vi "main.vi"() -> ()   [LabVIEW 2024]
uses:
  Controls/Who.ctl
  Controls/StratagemRing.ctl
  Controls/StateMachineState.ctl
  Controls/GameInfo.ctl
  Controls/E_Phases.ctl
  <vilib>/Platform/browser.llb/Open URL in Default Browser (string).vi
panel:
  in  "LastGame":bool
  in  "End Game":bool
  in  "Stratagems":T1 {"Cost" items=[" 1 CP", " 1 CP", " 2 CP", " 0 CP"]; "Name" items=["Command Reroll", " Smoke", " Fire and Fade", " Not in Data"]}
  in  "Spend2":bool
  in  "Spend1":bool
  in  "StratList":bool
  out "Wiki":string="Feeling lost? Click me to use Wiki "
  in  "DiscardM2":bool
  in  "DiscardM1":bool
  in  "Mission 2":dbl
  in  "Mission 1":dbl
  out "Victory points":dbl
  in  "Scored Primary":dbl
  out "BattleRound":dbl
  out "Command Points":dbl
  out "DidIStart?":bool
  in  "Who is going first?":T2
  out "Phase":string
  in  "GainCP":bool
  in  "NextPhase":bool
  in  "StartGame":bool
  out "error out":errorcluster
  in  "error in":errorcluster
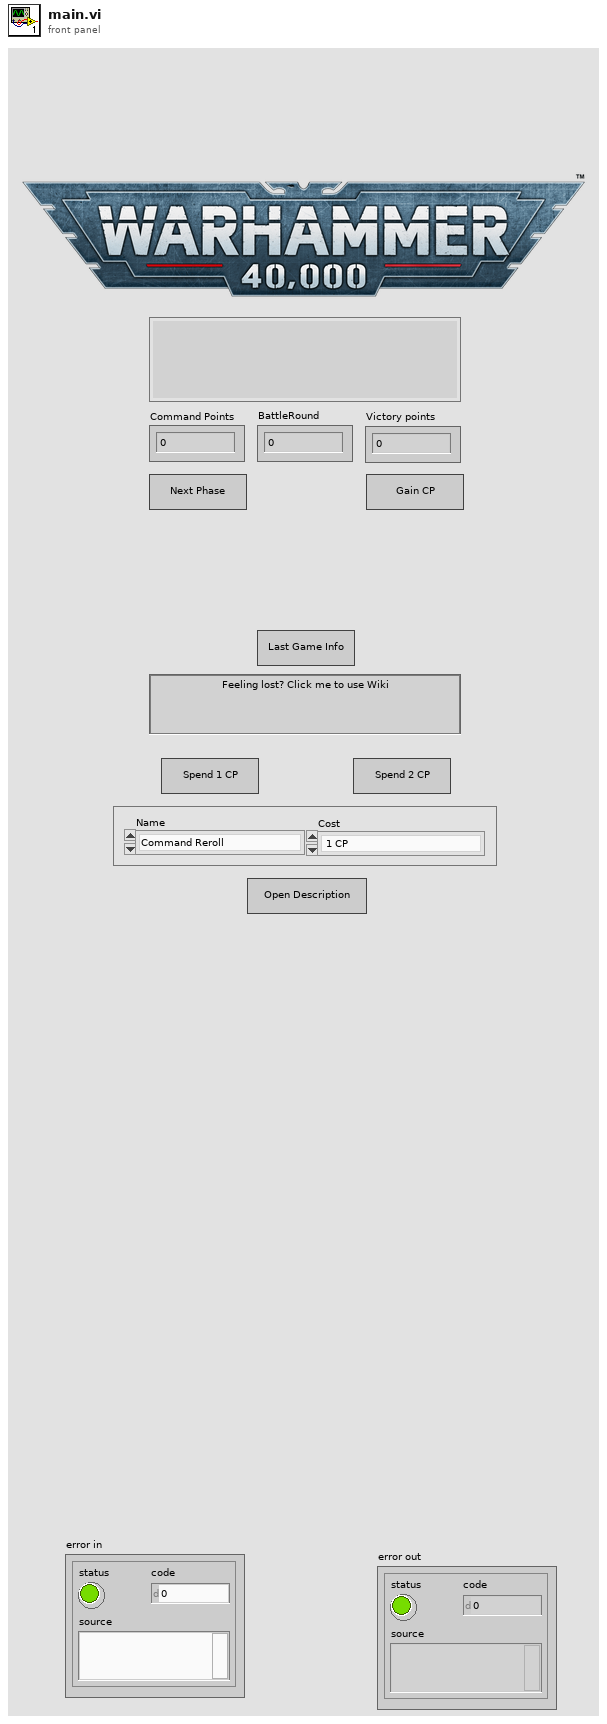
[diagram p1: front panel]
types:
  T1 = typedef "StratagemRing.ctl" = cluster{"Name":u16, "Cost":u16}
  T2 = typedef "Who.ctl" = enum16{"Me", "Opponent"}
  T3 = typedef "GameInfo.ctl" = cluster{"Player":string, "Opponent":string, "PArmy":string, "OArmy":string, "CP":dbl, "VP":dbl, "GameStart":timestamp, "GameEnd":timestamp, "BattleRound":dbl, "PrimaryMissionPoints":dbl, "SecondaryMissionPoints":dbl, "BattlePhase":T4, "Win":dbl, "Lose":dbl}
  T4 = typedef "E_Phases.ctl" = enum16{"Null/Error", "Command Phase", "Movement Phase", "Shooting Phase", "Charge Phase", "Fight Phase", "Secondary Scoring", "Enemy Command Phase", "Enemy Movement Phase", "Enemy Shooting Phase", "Enemy Charge Phase", "Enemy Fight Phase", "Enemy Secondary Scoring"}
  T5 = typedef "StateMachineState.ctl" = enum16{"Application Error", "Init", "Idle", "DataAnalysis", "Save", "Stop", "Error Handling"}
  T6 = enum8{"Enabled", "Disabled", "Disabled and Grayed Out"}
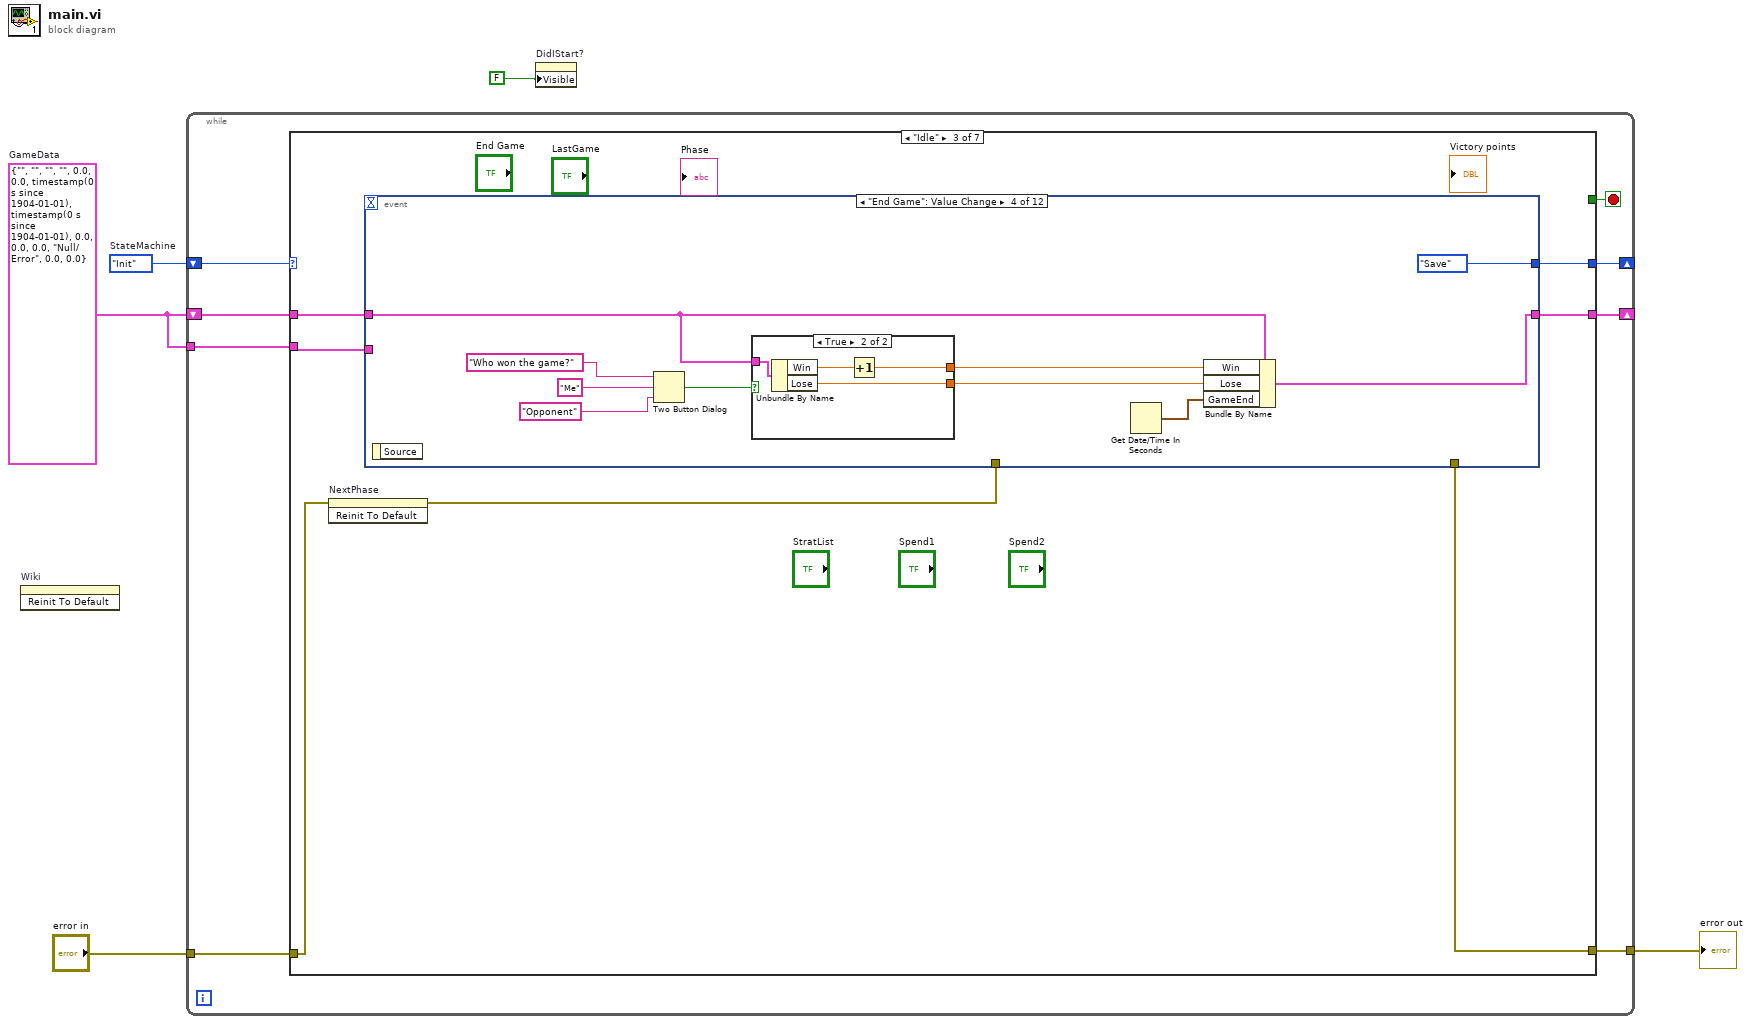
[diagram p0: block diagram]
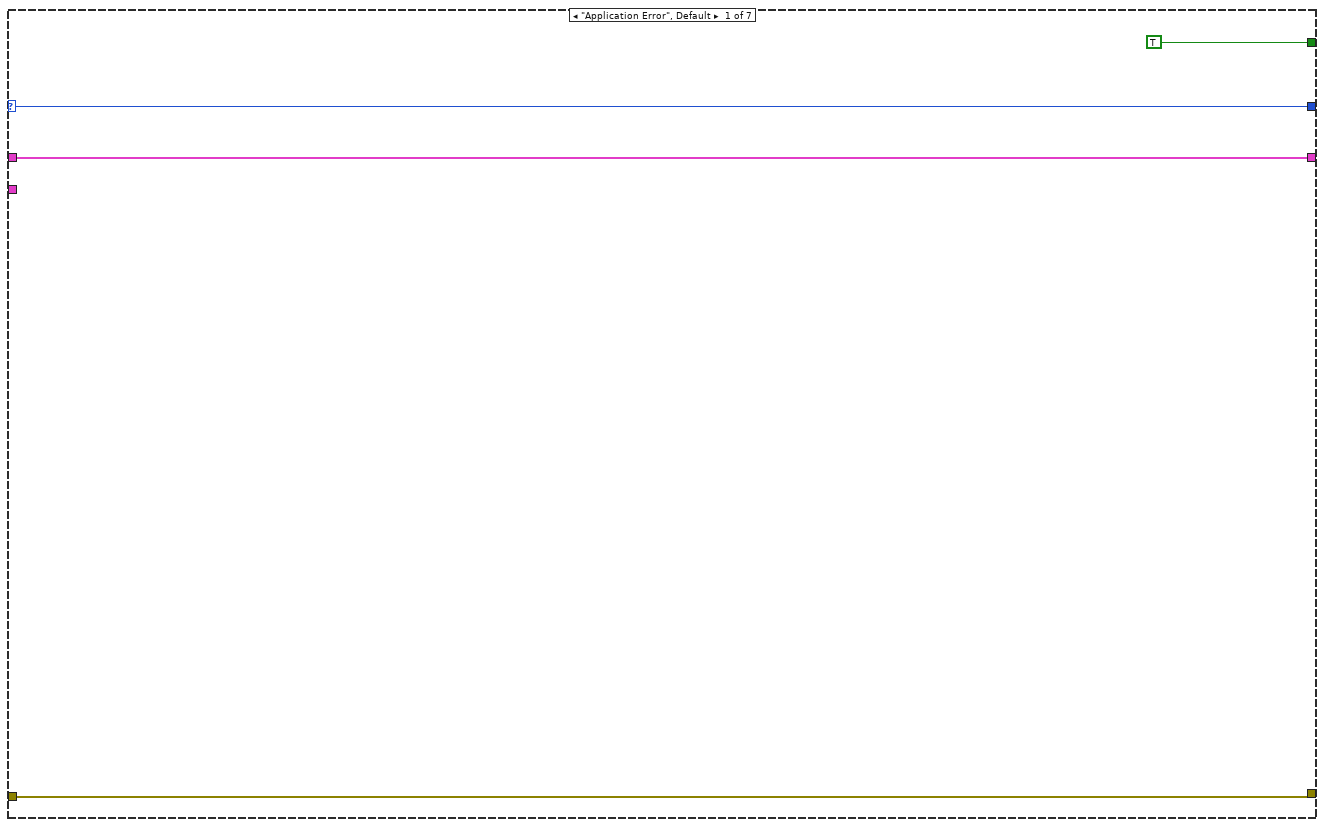
[diagram p2: hidden frame]
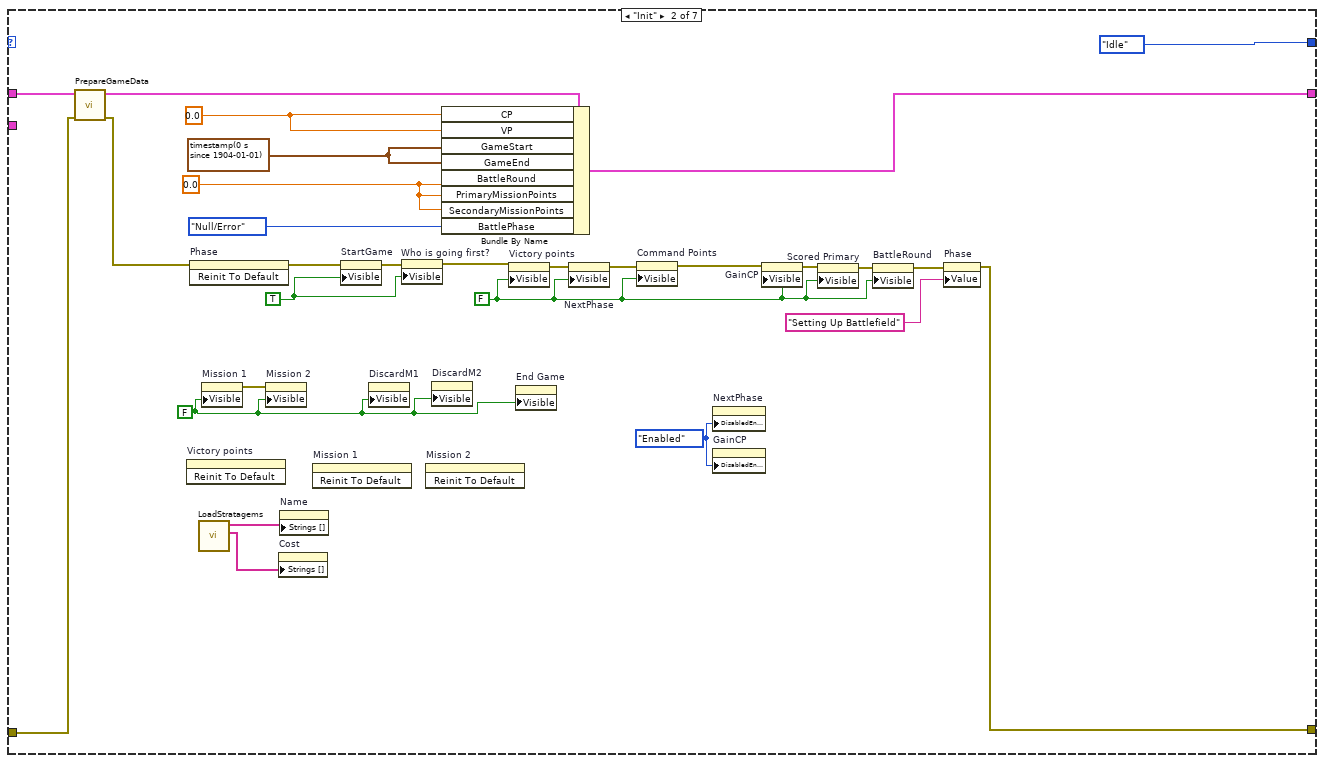
[diagram p3: hidden frame]
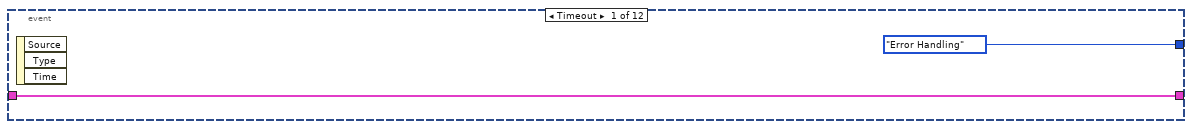
[diagram p4: hidden frame]
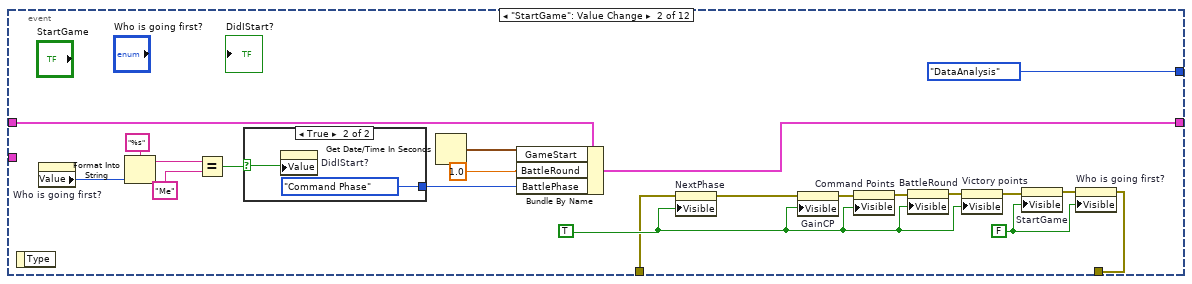
[diagram p5: hidden frame]
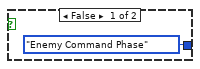
[diagram p6: hidden frame]
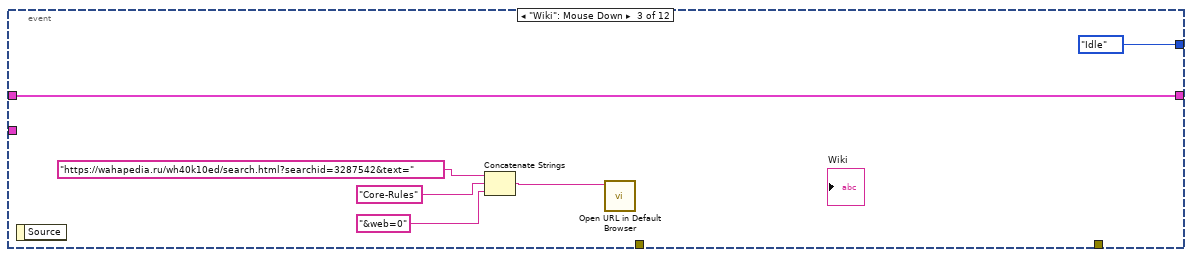
[diagram p7: hidden frame]
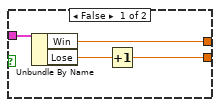
[diagram p8: hidden frame]
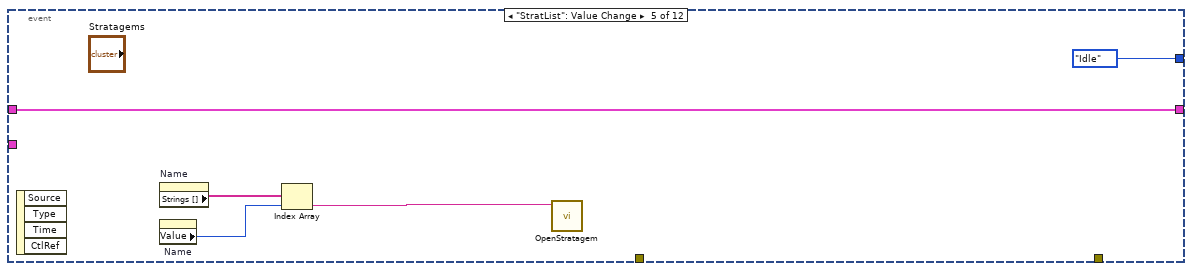
[diagram p9: hidden frame]
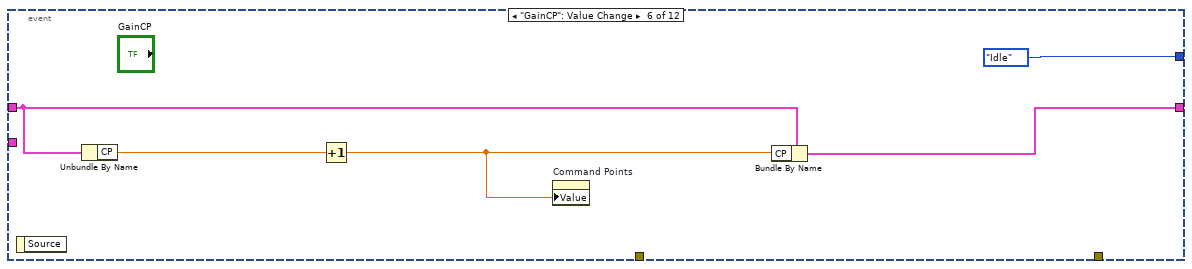
[diagram p10: hidden frame]
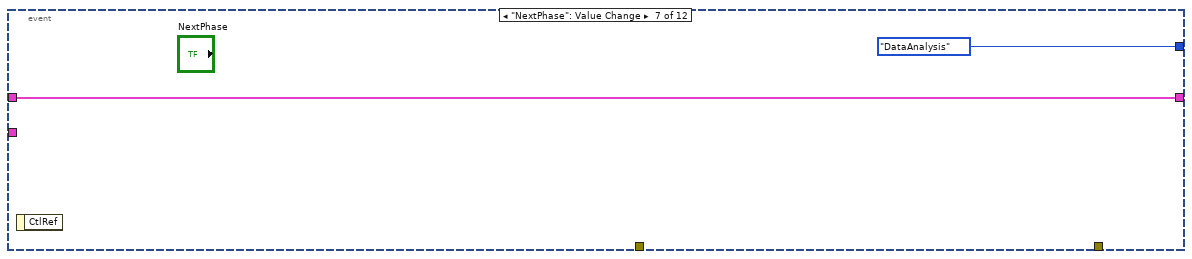
[diagram p11: hidden frame]
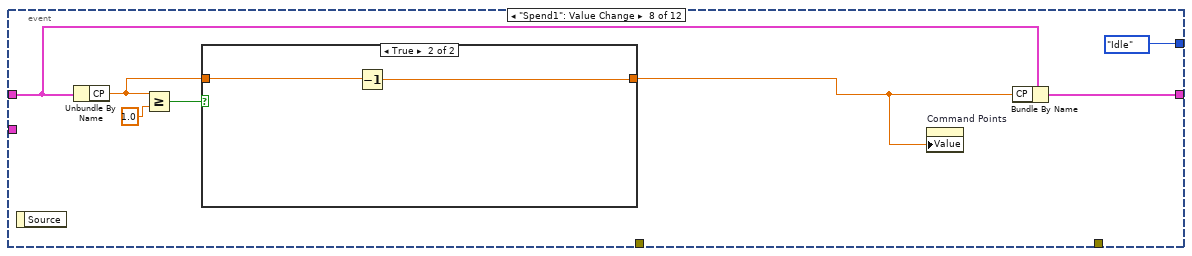
[diagram p12: hidden frame]
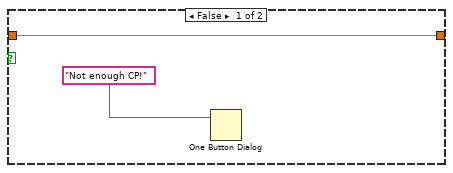
[diagram p13: hidden frame]
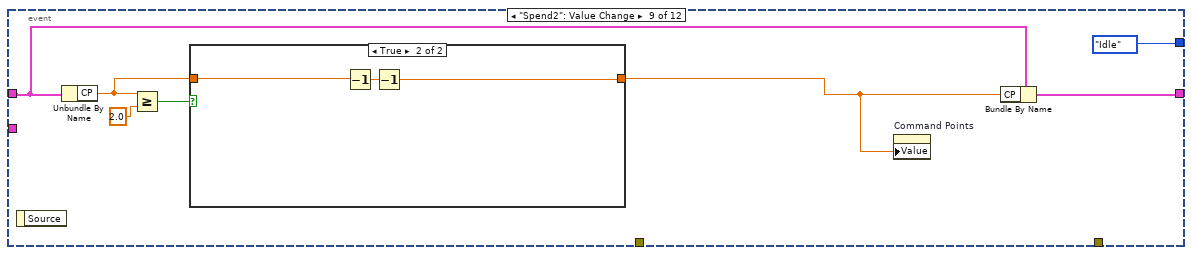
[diagram p14: hidden frame]
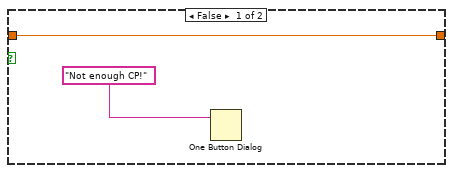
[diagram p15: hidden frame]
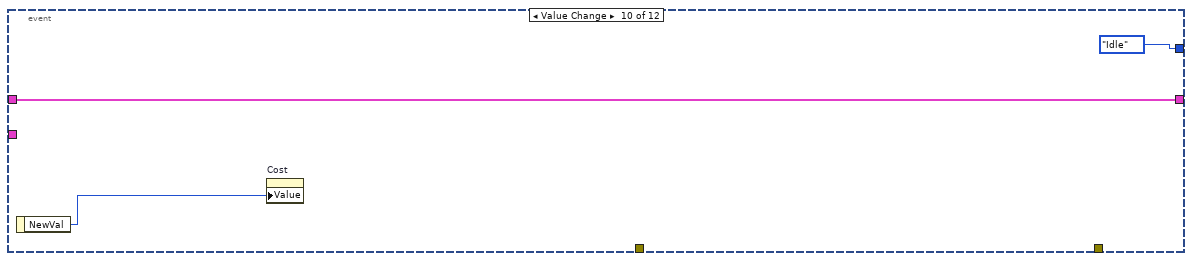
[diagram p16: hidden frame]
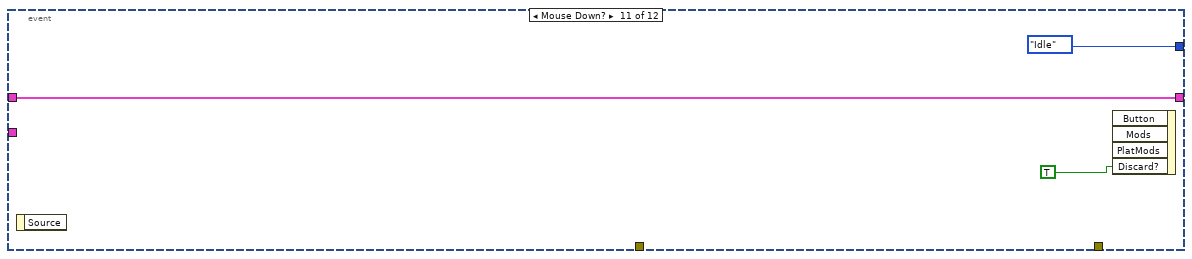
[diagram p17: hidden frame]
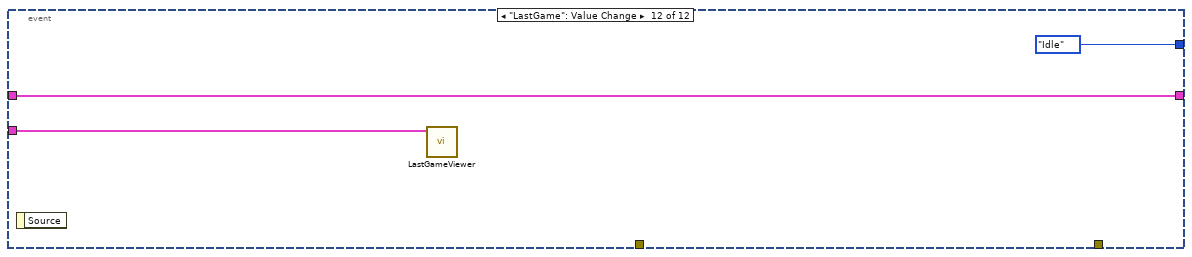
[diagram p18: hidden frame]
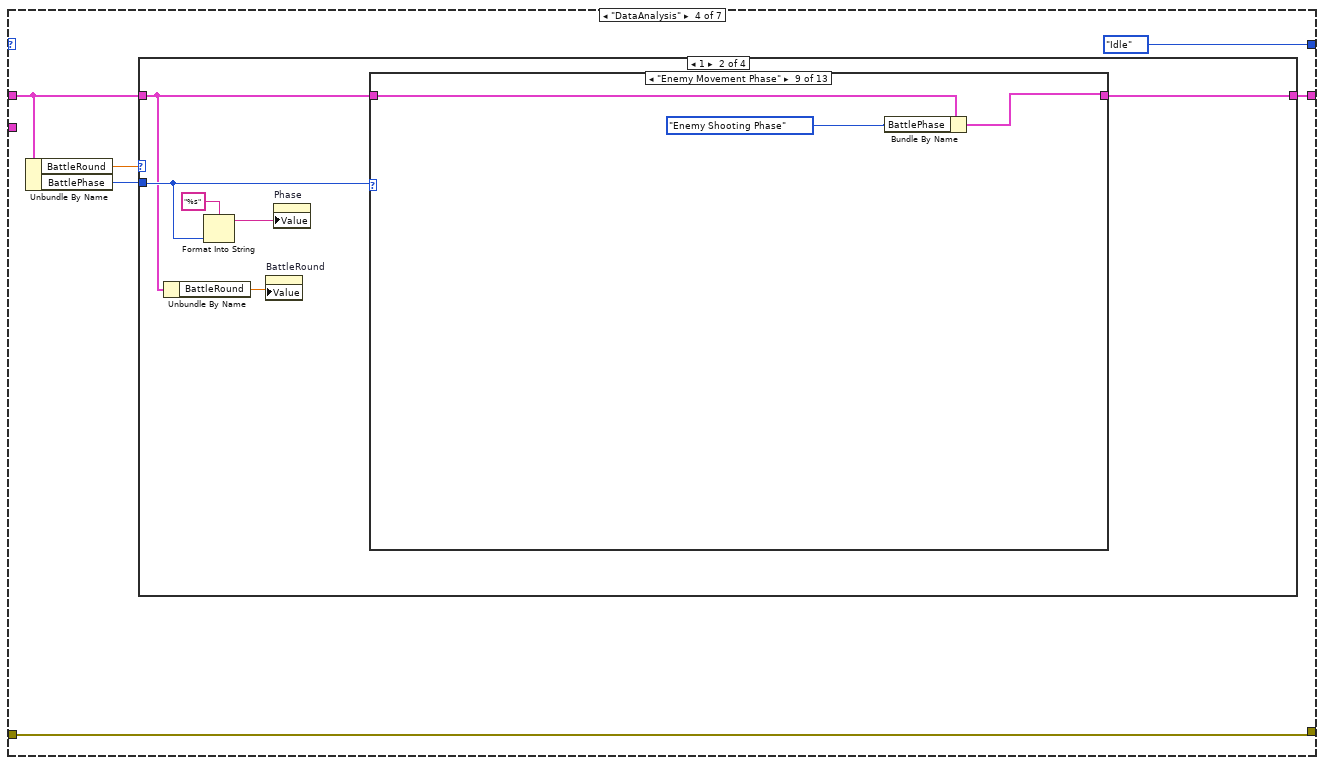
[diagram p19: hidden frame]
diagram:
  w1 = T3 {"Player"="", "Opponent"="", "PArmy"="", "OArmy"="", "CP"=0.0, "VP"=0.0, "GameStart"=timestamp(0 s since 1904-01-01), "GameEnd"=timestamp(0 s since 1904-01-01), "BattleRound"=0.0, "PrimaryMissionPoints"=0.0, "SecondaryMissionPoints"=0.0, "BattlePhase"=enum."Null/Error", "Win"=0.0, "Lose"=0.0}  # GameData
  w5 = StateMachineState."Init"  # StateMachine
  n1 = invoke on="Wiki" class="Str" method="Reinit To Default"() -> ()  [unwired: 3 in, 3 out]
  n2 = while {
    shift-right: [w11] -> _
    shift-left: w5 -> [w13]
    shift-right: [w9] -> _
    shift-left: w1 -> [w7]
    tunnel: "error in" -> [w10]
    tunnel: [w8] -> w3
    tunnel: w1 -> [w6]
    stop <- w12 stop-if-true
    n3 = case shown="\"Idle\"" w13 {
      selector: w13 -> [w16 _ _ _ _ _ _]
      tunnel: [TRUE _ _ _ _ TRUE _] -> w12
      tunnel: [w16 StateMachineState."Idle" ("StateMachine") w50 StateMachineState."Idle" ("StateMachine") StateMachineState."Stop" ("StateMachine") _ StateMachineState."Application Error" ("StateMachine")] -> w11
      tunnel: w7 -> [w15 w44 w52 w148 w378 w383 w386]
      tunnel: w10 -> [w14 w45 w49 w151 w379 w381 w384]
      tunnel: [w15 w39 w51 w147 w378 w383 w386] -> w9
      tunnel: [w14 w37 w48 w151 w379 w381 w384] -> w8
      tunnel: w6 -> [_ _ w46 _ _ _ _]
      frame "Application Error", Default {
      }
      frame "Init" {
        w19 = T6."Enabled" ("Disabled")
        w20 = FALSE ("Visible")
        w26 = FALSE ("Visible")
        w33 = TRUE ("Visible")
        w41 = 0.0 ("BattleRound")
        w42 = 0.0 ("VP")
        w38 = timestamp(0 s since 1904-01-01) ("GameEnd")
        n4 = call "PrepareGameData.vi"("error in"=w45, "GameDataIn"=w44) -> ("error out"=w18:errorcluster, "GameDataOut"=w43:T3)  [unwired: 8 in]
        n5 = invoke on="Victory points" class="DigNum (strict)" method="Reinit To Default"() -> ()  [unwired: 3 in, 3 out]
        n6 = invoke on="Phase" class="Str" method="Reinit To Default"(error in=w18) -> (error out=w35:errorcluster)  [unwired: 2 in, 2 out]
        n7 = call "LoadStratagems.vi"() -> ("Array"=w22:string[], "Array 2"=w21:string[])  [unwired: 9 in, 1 out]
        n8 = property on="Mission 1" class="DigNum (strict)"("Visible"=w20) -> (error out=w23:errorcluster)  [unwired: 2 in, 1 out]
        n9 = property on="Mission 2" class="DigNum (strict)"(error in=w23, "Visible"=w20) -> ()  [unwired: 1 in, 2 out]
        n10 = property on="Cost" class="Ring (strict)"("Strings []"=w22) -> ()  [unwired: 2 in, 2 out]
        n11 = property on="Name" class="Ring (strict)"("Strings []"=w21) -> ()  [unwired: 2 in, 2 out]
        n12 = invoke on="Mission 1" class="DigNum (strict)" method="Reinit To Default"() -> ()  [unwired: 3 in, 3 out]
        n13 = property on="StartGame" class="Bool"(error in=w35, "Visible"=w33) -> (error out=w32:errorcluster)  [unwired: 1 in, 1 out]
        n14 = property on="DiscardM1" class="Bool"("Visible"=w20) -> ()  [unwired: 2 in, 2 out]
        n15 = property on="Who is going first?" class="Enum (strict)"(error in=w32, "Visible"=w33) -> (error out=w25:errorcluster)  [unwired: 1 in, 1 out]
        n16 = invoke on="Mission 2" class="DigNum (strict)" method="Reinit To Default"() -> ()  [unwired: 3 in, 3 out]
        n17 = property on="DiscardM2" class="Bool"("Visible"=w20) -> ()  [unwired: 2 in, 2 out]
        n18 = Bundle By Name(cluster=w43, "CP"=w42, "VP"=w42, "GameStart"=w38, "GameEnd"=w38, "BattleRound"=w41, "PrimaryMissionPoints"=w41, "SecondaryMissionPoints"=w41, "BattlePhase"=E_Phases."Null/Error") -> (w39:T3)
        n19 = property on="Victory points" class="DigNum (strict)"(error in=w25, "Visible"=w26) -> (error out=w27:errorcluster)  [unwired: 1 in, 1 out]
        n20 = property on="End Game" class="Bool"("Visible"=w20) -> ()  [unwired: 2 in, 2 out]
        n21 = property on="NextPhase" class="Bool"(error in=w27, "Visible"=w26) -> (error out=w31:errorcluster)  [unwired: 1 in, 1 out]
        n22 = property on="Command Points" class="DigNum (strict)"(error in=w31, "Visible"=w26) -> (error out=w24:errorcluster)  [unwired: 1 in, 1 out]
        n23 = property on="NextPhase" class="Bool"("DisabledEnum"=w19) -> ()  [unwired: 2 in, 2 out]
        n24 = property on="GainCP" class="Bool"("DisabledEnum"=w19) -> ()  [unwired: 2 in, 2 out]
        n25 = property on="GainCP" class="Bool"(error in=w24, "Visible"=w26) -> (error out=w30:errorcluster)  [unwired: 1 in, 1 out]
        n26 = property on="Scored Primary" class="DigNum (strict)"(error in=w30, "Visible"=w26) -> (error out=w29:errorcluster)  [unwired: 1 in, 1 out]
        n27 = property on="BattleRound" class="DigNum (strict)"(error in=w29, "Visible"=w26) -> (error out=w28:errorcluster)  [unwired: 1 in, 1 out]
        n28 = property on="Phase" class="Str"(error in=w28, "Value"="Setting Up Battlefield" ("Phase")) -> (error out=w37:errorcluster)  [unwired: 1 in, 1 out]
      }
      frame "Idle" {
        n29 = invoke on="NextPhase" class="Bool" method="Reinit To Default"(error in=w49) -> (error out=w47:errorcluster)  [unwired: 2 in, 2 out]
        n30 = event shown="[3] \"End Game\": Value Change" {
          selector: _ -> [_ _ _ _ _ _ _ _ _ _ _ _]
          dyn-events: _ -> [_ _ _ _ _ _ _ _ _ _ _ _]
          timeout: _ -> [_ _ _ _ _ _ _ _ _ _ _ _]
          tunnel: w52 -> [w53 w75 w79 w85 w103 w111 w114 w119 w129 w140 w141 w146]
          tunnel: [w53 w73 w79 w86 w103 w112 w114 w116 w128 w140 w141 w146] -> w51
          tunnel: [StateMachineState."Error Handling" ("StateMachine") StateMachineState."DataAnalysis" ("StateMachine") StateMachineState."Idle" ("StateMachine") StateMachineState."Save" ("StateMachine") StateMachineState."Idle" ("StateMachine") StateMachineState."Idle" ("StateMachine") StateMachineState."DataAnalysis" ("StateMachine") StateMachineState."Idle" ("StateMachine") StateMachineState."Idle" ("StateMachine") StateMachineState."Idle" ("StateMachine") StateMachineState."Idle" ("StateMachine") StateMachineState."Idle" ("StateMachine")] -> w50
          tunnel: [_ w61 _ _ _ _ _ _ _ _ _ _] -> w48
          tunnel: w47 -> [_ w55 _ _ _ _ _ _ _ _ _ _]
          tunnel: w46 -> [_ _ _ _ _ _ _ _ _ _ _ w145]
          event Timeout {
            n31 = event-data() -> ()  [unwired: 1 in, 3 out]
          }
          event "StartGame": Value Change {
            w63 = FALSE ("Visible")
            w58 = TRUE ("Visible")
            n32 = event-data() -> ()  [unwired: 1 in, 1 out]
            n33 = property on="Who is going first?" class="Enum (strict)"() -> ("Value"=w70:T2)  [unwired: 2 in, 2 out]
            n34 = Format Into String(format string="%s", w70) -> (resulting string=w68:string)  [unwired: 2 in, 1 out]
            n35 = Equal?(x=w68, y="Me") -> (x = y?=w66:bool)
            n36 = case shown="True" w66 {
              selector: w66 -> [_ w77]
              tunnel: [E_Phases."Enemy Command Phase" ("BattlePhase") E_Phases."Command Phase" ("BattlePhase")] -> w65
              frame False {
              }
              frame True {
                n37 = property on="DidIStart?" class="Bool (strict)"("Value"=w77) -> ()  [unwired: 2 in, 2 out]
              }
            }
            n38 = Get Date/Time In Seconds() -> (seconds since 1Jan1904=w74:timestamp)
            n39 = Bundle By Name(cluster=w75, "GameStart"=w74, "BattleRound"=1.0, "BattlePhase"=w65) -> (w73:T3)
            n40 = property on="NextPhase" class="Bool"(error in=w55, "Visible"=w58) -> (error out=w56:errorcluster)  [unwired: 1 in, 1 out]
            n41 = property on="GainCP" class="Bool"(error in=w56, "Visible"=w58) -> (error out=w62:errorcluster)  [unwired: 1 in, 1 out]
            n42 = property on="Command Points" class="DigNum (strict)"(error in=w62, "Visible"=w58) -> (error out=w60:errorcluster)  [unwired: 1 in, 1 out]
            n43 = property on="BattleRound" class="DigNum (strict)"(error in=w60, "Visible"=w58) -> (error out=w59:errorcluster)  [unwired: 1 in, 1 out]
            n44 = property on="Victory points" class="DigNum (strict)"(error in=w59, "Visible"=w58) -> (error out=w57:errorcluster)  [unwired: 1 in, 1 out]
            n45 = property on="StartGame" class="Bool"(error in=w57, "Visible"=w63) -> (error out=w64:errorcluster)  [unwired: 1 in, 1 out]
            n46 = property on="Who is going first?" class="Enum (strict)"(error in=w64, "Visible"=w63) -> (error out=w61:errorcluster)  [unwired: 1 in, 1 out]
          }
          event "Wiki": Mouse Down {
            n47 = event-data() -> ()  [unwired: 1 in, 1 out]
            n48 = Concatenate Strings("https://wahapedia.ru/wh40k10ed/search.html?searchid=3287542&text=" ("string"), "Core-Rules" ("string"), "&web=0" ("string")) -> (w84:string)
            n49 = call-poly <vilib>:"Open URL in Default Browser.vi"("URL"=w84) -> ()  [unwired: 5 in, 2 out]
          }
          event "End Game": Value Change {
            n50 = event-data() -> ()  [unwired: 1 in, 1 out]
            n51 = Two Button Dialog(message="Who won the game?", 1:"Opponent" ("F button name (\"Cancel\")"), 2:"Me" ("T button name (\"OK\")")) -> (T button?=w90:bool)
            n52 = case shown="True" w90 {
              tunnel: w85 -> [w98 w102]
              tunnel: [w96 w100] -> w88
              tunnel: [w97 w99] -> w87
              frame False {
                n53 = Unbundle By Name(w98) -> ("Win"=w96:dbl, "Lose"=w95:dbl)
                n54 = Increment(x=w95) -> (x+1=w97:dbl)
              }
              frame True {
                n55 = Unbundle By Name(w102) -> ("Win"=w101:dbl, "Lose"=w99:dbl)
                n56 = Increment(x=w101) -> (x+1=w100:dbl)
              }
            }
            n57 = Get Date/Time In Seconds() -> (seconds since 1Jan1904=w89:timestamp)
            n58 = Bundle By Name(cluster=w85, "Win"=w88, "Lose"=w87, "GameEnd"=w89) -> (w86:T3)
          }
          event "StratList": Value Change {
            n59 = event-data() -> ()  [unwired: 1 in, 4 out]
            n60 = property on="Name" class="Ring (strict)"() -> ("Strings []"=w106:string[])  [unwired: 2 in, 2 out]
            n61 = property on="Name" class="Ring (strict)"() -> ("Value"=w105:u16)  [unwired: 2 in, 2 out]
            n62 = Index Array(array=w106, index=w105) -> (element=w104:string)
            n63 = call "OpenStratagem.vi"("String"=w104) -> ()  [unwired: 11 in]
          }
          event "GainCP": Value Change {
            n64 = event-data() -> ()  [unwired: 1 in, 1 out]
            n65 = Unbundle By Name(w111) -> ("CP"=w110:dbl)
            n66 = Increment(x=w110) -> (x+1=w108:dbl)
            n67 = property on="Command Points" class="DigNum (strict)"("Value"=w108) -> ()  [unwired: 2 in, 2 out]
            n68 = Bundle By Name(cluster=w111, "CP"=w108) -> (w112:T3)
          }
          event "NextPhase": Value Change {
            n69 = event-data() -> ()  [unwired: 1 in, 1 out]
          }
          event "Spend1": Value Change {
            n70 = event-data() -> ()  [unwired: 1 in, 1 out]
            n71 = Unbundle By Name(w119) -> ("CP"=w118:dbl)
            n72 = Greater Or Equal?(x=w118, y=1.0) -> (x >= y?=w120:bool)
            n73 = case shown="True" w120 {
              tunnel: w118 -> [w123 w125]
              tunnel: [w123 w124] -> w115
              frame False {
                n74 = One Button Dialog(message="Not enough CP!") -> ()  [unwired: 1 in, 1 out]
              }
              frame True {
                n75 = Decrement(x=w125) -> (x-1=w124:dbl)
              }
            }
            n76 = property on="Command Points" class="DigNum (strict)"("Value"=w115) -> ()  [unwired: 2 in, 2 out]
            n77 = Bundle By Name(cluster=w119, "CP"=w115) -> (w116:T3)
          }
          event "Spend2": Value Change {
            n78 = event-data() -> ()  [unwired: 1 in, 1 out]
            n79 = Unbundle By Name(w129) -> ("CP"=w130:dbl)
            n80 = Greater Or Equal?(x=w130, y=2.0) -> (x >= y?=w131:bool)
            n81 = case shown="True" w131 {
              tunnel: w130 -> [w134 w137]
              tunnel: [w134 w135] -> w126
              frame False {
                n82 = One Button Dialog(message="Not enough CP!") -> ()  [unwired: 1 in, 1 out]
              }
              frame True {
                n83 = Decrement(x=w137) -> (x-1=w136:dbl)
                n84 = Decrement(x=w136) -> (x-1=w135:dbl)
              }
            }
            n85 = property on="Command Points" class="DigNum (strict)"("Value"=w126) -> ()  [unwired: 2 in, 2 out]
            n86 = Bundle By Name(cluster=w129, "CP"=w126) -> (w128:T3)
          }
          event Value Change {
            n87 = event-data() -> ("NewVal"=w138:u16)  [unwired: 1 in]
            n88 = property on="Cost" class="Ring (strict)"("Value"=w138) -> ()  [unwired: 2 in, 2 out]
          }
          event Mouse Down? {
            n89 = event-data() -> ()  [unwired: 1 in, 1 out]
            n90 = event-data("Discard?"=TRUE) -> ()  [unwired: 4 in, 1 out]
          }
          event "LastGame": Value Change {
            n91 = event-data() -> ()  [unwired: 1 in, 1 out]
            n92 = call "LastGameViewer.vi"("GameData"=w145) -> ()  [unwired: 11 in]
          }
        }
      }
      frame "DataAnalysis" {
        n93 = Unbundle By Name(w148) -> ("BattleRound"=w150:dbl, "BattlePhase"=w149:T4)
        n94 = case shown="1" w150 {
          tunnel: w149 -> [_ w156 w229 _]
          tunnel: w148 -> [w153 w155 w228 w319]
          tunnel: [w153 w159 w232 w319] -> w147
          frame 0, Default {
          }
          frame 1 {
            n95 = Unbundle By Name(w155) -> ("BattleRound"=w154:dbl)
            n96 = Format Into String(format string="%s", w156) -> (resulting string=w158:string)  [unwired: 2 in, 1 out]
            n97 = property on="BattleRound" class="DigNum (strict)"("Value"=w154) -> ()  [unwired: 2 in, 2 out]
            n98 = property on="Phase" class="Str"("Value"=w158) -> ()  [unwired: 2 in, 2 out]
            n99 = case shown="\"Enemy Movement Phase\"" w156 {
              tunnel: w155 -> [w160 w164 w167 w170 w173 w176 w184 w195 w199 w202 w205 w208 w211]
              tunnel: [w160 w165 w168 w171 w174 w177 w186 w197 w200 w203 w206 w209 w212] -> w159
              frame "Null/Error", Default {
              }
              frame "Command Phase" {
                n100 = Unbundle By Name(w164) -> ("CP"=w163:dbl)
                n101 = Increment(x=w163) -> (x+1=w161:dbl)
                n102 = property on="Command Points" class="DigNum (strict)"("Value"=w161) -> ()  [unwired: 2 in, 2 out]
                n103 = Bundle By Name(cluster=w164, "CP"=w161, "BattlePhase"=E_Phases."Movement Phase") -> (w165:T3)
              }
              frame "Movement Phase" {
                n104 = Bundle By Name(cluster=w167, "BattlePhase"=E_Phases."Shooting Phase") -> (w168:T3)
              }
              frame "Shooting Phase" {
                n105 = Bundle By Name(cluster=w170, "BattlePhase"=E_Phases."Charge Phase") -> (w171:T3)
              }
              frame "Charge Phase" {
                n106 = Bundle By Name(cluster=w173, "BattlePhase"=E_Phases."Fight Phase") -> (w174:T3)
              }
              frame "Fight Phase" {
                n107 = Bundle By Name(cluster=w176, "BattlePhase"=E_Phases."Secondary Scoring") -> (w177:T3)
              }
              frame "Secondary Scoring" {
                n108 = Unbundle By Name(w184) -> ("VP"=w180:dbl, "PrimaryMissionPoints"=w181:dbl, "SecondaryMissionPoints"=w182:dbl, "BattleRound"=w178:dbl)
                n109 = property on="DidIStart?" class="Bool (strict)"() -> ("Value"=w185:bool)  [unwired: 2 in, 2 out]
                n110 = property on="BattleRound" class="DigNum (strict)"("Value"=w178) -> ()  [unwired: 2 in, 2 out]
                n111 = case shown="False" w185 {
                  tunnel: w178 -> [w190 w191]
                  tunnel: [E_Phases."Enemy Command Phase" ("BattlePhase") E_Phases."Enemy Command Phase" ("BattlePhase")] -> w183
                  tunnel: [w189 w191] -> w179
                  frame False {
                    n112 = Increment(x=w190) -> (x+1=w189:dbl)
                    n113 = property on="DidIStart?" class="Bool (strict)"("Value"=TRUE ("Boolean")) -> ()  [unwired: 2 in, 2 out]
                  }
                  frame True {
                    n114 = property on="DidIStart?" class="Bool (strict)"("Value"=FALSE ("Boolean")) -> ()  [unwired: 2 in, 2 out]
                  }
                }
                n115 = Bundle By Name(cluster=w184, "VP"=w180, "PrimaryMissionPoints"=w181, "SecondaryMissionPoints"=w182, "BattleRound"=w179, "BattlePhase"=w183) -> (w186:T3)
              }
              frame "Enemy Command Phase" {
                n116 = Unbundle By Name(w195) -> ("CP"=w196:dbl)
                n117 = Increment(x=w196) -> (x+1=w194:dbl)
                n118 = property on="Command Points" class="DigNum (strict)"("Value"=w194) -> ()  [unwired: 2 in, 2 out]
                n119 = Bundle By Name(cluster=w195, "CP"=w194, "BattlePhase"=E_Phases."Enemy Movement Phase") -> (w197:T3)
              }
              frame "Enemy Movement Phase" {
                n120 = Bundle By Name(cluster=w199, "BattlePhase"=E_Phases."Enemy Shooting Phase") -> (w200:T3)
              }
              frame "Enemy Shooting Phase" {
                n121 = Bundle By Name(cluster=w202, "BattlePhase"=E_Phases."Enemy Charge Phase") -> (w203:T3)
              }
              frame "Enemy Charge Phase" {
                n122 = Bundle By Name(cluster=w205, "BattlePhase"=E_Phases."Enemy Fight Phase") -> (w206:T3)
              }
              frame "Enemy Fight Phase" {
                n123 = Bundle By Name(cluster=w208, "BattlePhase"=E_Phases."Enemy Secondary Scoring") -> (w209:T3)
              }
              frame "Enemy Secondary Scoring" {
                n124 = Unbundle By Name(w211) -> ("VP"=w216:dbl, "PrimaryMissionPoints"=w217:dbl, "SecondaryMissionPoints"=w218:dbl, "BattleRound"=w219:dbl)
                n125 = property on="DidIStart?" class="Bool (strict)"() -> ("Value"=w214:bool)  [unwired: 2 in, 2 out]
                n126 = case shown="False" w214 {
                  tunnel: w219 -> [w221 w224]
                  tunnel: [E_Phases."Command Phase" ("BattlePhase") E_Phases."Command Phase" ("BattlePhase")] -> w213
                  tunnel: [w220 w224] -> w215
                  frame False {
                    n127 = Increment(x=w221) -> (x+1=w220:dbl)
                    n128 = property on="DidIStart?" class="Bool (strict)"("Value"=TRUE ("Boolean")) -> ()  [unwired: 2 in, 2 out]
                  }
                  frame True {
                    n129 = property on="DidIStart?" class="Bool (strict)"("Value"=FALSE ("Boolean")) -> ()  [unwired: 2 in, 2 out]
                  }
                }
                n130 = Bundle By Name(cluster=w211, "VP"=w216, "PrimaryMissionPoints"=w217, "SecondaryMissionPoints"=w218, "BattleRound"=w215, "BattlePhase"=w213) -> (w212:T3)
              }
            }
          }
          frame 2..5 {
            n131 = Unbundle By Name(w228) -> ("BattleRound"=w227:dbl)
            n132 = Format Into String(format string="%s", w229) -> (resulting string=w231:string)  [unwired: 2 in, 1 out]
            n133 = property on="BattleRound" class="DigNum (strict)"("Value"=w227) -> ()  [unwired: 2 in, 2 out]
            n134 = property on="Phase" class="Str"("Value"=w231) -> ()  [unwired: 2 in, 2 out]
            n135 = case shown="\"Enemy Secondary Scoring\"" w229 {
              tunnel: w228 -> [w233 w238 w245 w250 w253 w256 w265 w285 w289 w292 w295 w298 w302]
              tunnel: [w233 w239 w248 w251 w254 w257 w267 w287 w290 w293 w296 w299 w303] -> w232
              frame "Null/Error", Default {
              }
              frame "Command Phase" {
                n136 = Unbundle By Name(w238) -> ("CP"=w237:dbl)
                n137 = Increment(x=w237) -> (x+1=w235:dbl)
                "Command Points" <- w235
                n138 = property on="Scored Primary" class="DigNum (strict)"("Visible"=TRUE) -> ()  [unwired: 2 in, 2 out]
                n139 = Bundle By Name(cluster=w238, "CP"=w235, "BattlePhase"=E_Phases."Movement Phase") -> (w239:T3)
              }
              frame "Movement Phase" {
                n140 = Unbundle By Name(w245) -> ("PrimaryMissionPoints"=w242:dbl, "VP"=w244:dbl)
                n141 = Add(x=w244, y="Scored Primary") -> (x+y=w240:dbl)
                n142 = Add(x=w242, y=w240) -> (x+y=w241:dbl)
                n143 = property on="Scored Primary" class="DigNum (strict)"("Visible"=FALSE) -> ()  [unwired: 2 in, 2 out]
                n144 = property on="Victory points" class="DigNum (strict)"("Value"=w240) -> ()  [unwired: 2 in, 2 out]
                n145 = invoke on="Scored Primary" class="DigNum (strict)" method="Reinit To Default"() -> ()  [unwired: 3 in, 3 out]
                n146 = Bundle By Name(cluster=w245, "BattlePhase"=E_Phases."Shooting Phase", "PrimaryMissionPoints"=w241, "VP"=w240) -> (w248:T3)
              }
              frame "Shooting Phase" {
                n147 = Bundle By Name(cluster=w250, "BattlePhase"=E_Phases."Charge Phase") -> (w251:T3)
              }
              frame "Charge Phase" {
                n148 = Bundle By Name(cluster=w253, "BattlePhase"=E_Phases."Fight Phase") -> (w254:T3)
              }
              frame "Fight Phase" {
                n149 = Bundle By Name(cluster=w256, "BattlePhase"=E_Phases."Secondary Scoring") -> (w257:T3)
              }
              frame "Secondary Scoring" {
                w258 = TRUE ("Visible")
                n150 = property on="Mission 2" class="DigNum (strict)"("Visible"=w258) -> ()  [unwired: 2 in, 2 out]
                n151 = Unbundle By Name(w265) -> ("VP"=w261:dbl, "PrimaryMissionPoints"=w262:dbl, "SecondaryMissionPoints"=w263:dbl, "BattleRound"=w260:dbl)
                n152 = property on="DidIStart?" class="Bool (strict)"() -> ("Value"=w266:bool)  [unwired: 2 in, 2 out]
                n153 = property on="Mission 1" class="DigNum (strict)"("Visible"=w258) -> ()  [unwired: 2 in, 2 out]
                n154 = case shown="False" w266 {
                  tunnel: w260 -> [w271 w272]
                  tunnel: [E_Phases."Enemy Command Phase" ("BattlePhase") E_Phases."Enemy Command Phase" ("BattlePhase")] -> w264
                  tunnel: [w270 w272] -> w259
                  frame False {
                    n155 = Increment(x=w271) -> (x+1=w270:dbl)
                    n156 = property on="DidIStart?" class="Bool (strict)"("Value"=TRUE ("Boolean")) -> ()  [unwired: 2 in, 2 out]
                  }
                  frame True {
                    n157 = property on="DidIStart?" class="Bool (strict)"("Value"=FALSE ("Boolean")) -> ()  [unwired: 2 in, 2 out]
                  }
                }
                n158 = Bundle By Name(cluster=w265, "VP"=w261, "PrimaryMissionPoints"=w262, "SecondaryMissionPoints"=w263, "BattleRound"=w259, "BattlePhase"=w264) -> (w267:T3)
              }
              frame "Enemy Command Phase" {
                w283 = FALSE ("Visible")
                n159 = Unbundle By Name(w285) -> ("CP"=w286:dbl, "VP"=w281:dbl, "SecondaryMissionPoints"=w278:dbl)
                n160 = property on="Mission 1" class="DigNum (strict)"("Visible"=w283) -> (error out=w282:errorcluster)  [unwired: 2 in, 1 out]
                n161 = property on="Mission 1" class="DigNum (strict)"() -> ("Value"=w279:dbl)  [unwired: 2 in, 2 out]
                n162 = property on="Mission 2" class="DigNum (strict)"() -> ("Value"=w280:dbl)  [unwired: 2 in, 2 out]
                n163 = property on="Mission 2" class="DigNum (strict)"(error in=w282, "Visible"=w283) -> ()  [unwired: 1 in, 2 out]
                n164 = Add(x=w279, y=w280) -> (x+y=w275:dbl)
                n165 = Increment(x=w286) -> (x+1=w284:dbl)
                n166 = invoke on="Mission 1" class="DigNum (strict)" method="Reinit To Default"() -> ()  [unwired: 3 in, 3 out]
                n167 = Add(x=w278, y=w275) -> (x+y=w277:dbl)
                n168 = property on="Command Points" class="DigNum (strict)"("Value"=w284) -> ()  [unwired: 2 in, 2 out]
                n169 = invoke on="Mission 2" class="DigNum (strict)" method="Reinit To Default"() -> ()  [unwired: 3 in, 3 out]
                n170 = Add(x=w281, y=w275) -> (x+y=w276:dbl)
                n171 = property on="Victory points" class="DigNum (strict)"("Value"=w276) -> ()  [unwired: 2 in, 2 out]
                n172 = Bundle By Name(cluster=w285, "CP"=w284, "BattlePhase"=E_Phases."Enemy Movement Phase", "VP"=w276, "SecondaryMissionPoints"=w277) -> (w287:T3)
              }
              frame "Enemy Movement Phase" {
                n173 = Bundle By Name(cluster=w289, "BattlePhase"=E_Phases."Enemy Shooting Phase") -> (w290:T3)
              }
              frame "Enemy Shooting Phase" {
                n174 = Bundle By Name(cluster=w292, "BattlePhase"=E_Phases."Enemy Charge Phase") -> (w293:T3)
              }
              frame "Enemy Charge Phase" {
                n175 = Bundle By Name(cluster=w295, "BattlePhase"=E_Phases."Enemy Fight Phase") -> (w296:T3)
              }
              frame "Enemy Fight Phase" {
                n176 = Bundle By Name(cluster=w298, "BattlePhase"=E_Phases."Enemy Secondary Scoring") -> (w299:T3)
              }
              frame "Enemy Secondary Scoring" {
                n177 = Unbundle By Name(w302) -> ("VP"=w306:dbl, "PrimaryMissionPoints"=w307:dbl, "SecondaryMissionPoints"=w308:dbl, "BattleRound"=w309:dbl)
                n178 = property on="DidIStart?" class="Bool (strict)"() -> ("Value"=w305:bool)  [unwired: 2 in, 2 out]
                n179 = case shown="True" w305 {
                  tunnel: w309 -> [w311 w314]
                  tunnel: [E_Phases."Command Phase" ("BattlePhase") E_Phases."Command Phase" ("BattlePhase")] -> w304
                  tunnel: [w310 w314] -> w301
                  frame False {
                    n180 = Increment(x=w311) -> (x+1=w310:dbl)
                    n181 = property on="DidIStart?" class="Bool (strict)"("Value"=TRUE ("Boolean")) -> ()  [unwired: 2 in, 2 out]
                  }
                  frame True {
                    n182 = property on="DidIStart?" class="Bool (strict)"("Value"=FALSE ("Boolean")) -> ()  [unwired: 2 in, 2 out]
                  }
                }
                n183 = Bundle By Name(cluster=w302, "VP"=w306, "PrimaryMissionPoints"=w307, "SecondaryMissionPoints"=w308, "BattleRound"=w301, "BattlePhase"=w304) -> (w303:T3)
              }
            }
          }
          frame 6 {
            w318 = T6."Disabled and Grayed Out" ("Disabled")
            n184 = property on="End Game" class="Bool"("Visible"=TRUE) -> ()  [unwired: 2 in, 2 out]
            n185 = property on="GainCP" class="Bool"("DisabledEnum"=w318) -> ()  [unwired: 2 in, 2 out]
            n186 = property on="NextPhase" class="Bool"("DisabledEnum"=w318) -> ()  [unwired: 2 in, 2 out]
          }
        }
      }
      frame "Save" {
        w332 = ""
        n187 = Unbundle By Name(w378) -> ("Player"=w375:string, "Win"=w369:dbl, "Lose"=w363:dbl, "GameStart"=w353:timestamp, "GameEnd"=w352:timestamp, "Opponent"=w351:string, "PArmy"=w350:string, "OArmy"=w349:string, "VP"=w342:dbl, "PrimaryMissionPoints"=w341:dbl, "SecondaryMissionPoints"=w340:dbl)
        n188 = Format Into String(format string="%d", w341) -> (resulting string=w338:string)  [unwired: 2 in, 1 out]
        n189 = Format Into String(format string="%d", w342) -> (resulting string=w337:string)  [unwired: 2 in, 1 out]
        n190 = Format Into String(format string="%d", w340) -> (resulting string=w339:string)  [unwired: 2 in, 1 out]
        n191 = Format Date/Time String(time format string (%c)="%B", seconds (now)=w353) -> (date/time string=w361:string)  [unwired: 1 in]
        n192 = Format Date/Time String(time format string (%c)="%d.%m.%Y - %H:%M", seconds (now)=w353) -> (date/time string=w358:string)  [unwired: 1 in]
        n193 = Format Date/Time String(time format string (%c)="%d.%m.%Y - %H:%M", seconds (now)=w352) -> (date/time string=w355:string)  [unwired: 1 in]
        n194 = Format Into String(format string="%d", w363) -> (resulting string=w365:string)  [unwired: 2 in, 1 out]
        n195 = Format Into String(format string="%d", w369) -> (resulting string=w368:string)  [unwired: 2 in, 1 out]
        n196 = Build Array("Victory Points" ("element"), w337) -> (w323:string[])
        n197 = Build Array("From Secondary" ("element"), w339) -> (w321:string[])
        n198 = Build Array("From Primary" ("element"), w338) -> (w322:string[])
        n199 = Build Array("Player Army" ("element"), w350) -> (w326:string[])
        n200 = Build Array("Opponent Army" ("element"), w349) -> (w325:string[])
        n201 = Build Array("Player" ("element"), w375) -> (w335:string[])
        n202 = Build Array("Opponent" ("element"), w351) -> (w327:string[])
        n203 = Build Array("Lose" ("element"), w365) -> (w333:string[])
        n204 = Build Array("Last Game Played" ("element"), w361) -> (w330:string[])
        n205 = Build Array("Start: " ("element"), w358) -> (w329:string[])
        n206 = Build Array("End: " ("element"), w355) -> (w328:string[])
        n207 = Build Array("Win" ("element"), w368) -> (w334:string[])
        n208 = Build Array(w332, w332) -> (w331:string[])
        n209 = Insert Into Array(array=string[][] [], new element #1=w335, new element #2=w334, new element #3=w333, new element #4=w331, new element #5=w330, new element #6=w329, new element #7=w328, new element #8=w327, new element #9=w326, new element #10=w325, new element #11=w323, new element #12=w322, new element #13=w321) -> (w324:string[][])  [unwired: 2 in]
        n210 = Array To Spreadsheet String(array=w324, 3:"%s" ("format string")) -> (spreadsheet string=w377:string)  [unwired: 1 in]
        n211 = Write to Text File(prompt (Choose or enter file path)="Where do You wanna save your Save File?", text=w377) -> ()  [unwired: 2 in, 3 out]
      }
      frame "Stop" {
      }
      frame "Error Handling" {
      }
    }
  }
  "error out" <- w3
  n212 = property on="DidIStart?" class="Bool (strict)"("Visible"=FALSE) -> ()  [unwired: 2 in, 2 out]
